vi "ElevatorCtrl_example.vi"() -> ()   [LabVIEW 2019]
uses:
  <vilib>/Rock Robotics/WPI/ThirdParty/JAS_Junk/TrajLib/TypeDef/LINEAR_SYSTEM_LOOP.ctl
  <vilib>/Rock Robotics/WPI/ThirdParty/JAS_Junk/TrajLib/TypeDef/LINEAR_QUADRATIC_REGULATOR.ctl
  <vilib>/Analysis/Matrix/Datatypes/RealMatrix.ctl
  <vilib>/Rock Robotics/WPI/ThirdParty/JAS_Junk/TrajLib/TypeDef/LINEAR_PLANT_INV_FF.ctl
  <vilib>/Rock Robotics/WPI/ThirdParty/JAS_Junk/TrajLib/TypeDef/KALMAN_FILTER.ctl
  <vilib>/Rock Robotics/WPI/ThirdParty/JAS_Junk/TrajLib/TypeDef/LINEAR_SYSTEM.ctl
  <vilib>/Rock Robotics/WPI/ThirdParty/JAS_Junk/TrajLib/Enum/DCMOTOR_TYPES_ENUM.ctl
  <vilib>/Rock Robotics/WPI/ThirdParty/JAS_Junk/TrajLib/BatterySim_CalculateLoadedBatteryVoltage.vi
  <vilib>/Rock Robotics/WPI/ThirdParty/JAS_Junk/TrajLib/Trajectory_Library.lvlib
  <vilib>/Analysis/Matrix/NI_Matrix.lvlib
panel:
  out "out Linear System Loop":T1
  out "Sim Error":bool
  in  "Tab Control":enum32{"Control"}(tab)
  out "Height Dmd \n(SP)":dbl format="%20.3f"
  out "Battery Voltage":dbl format="%20.3f"
  out "CO Chart":cluster{dbl, "Voltage":dbl}(graph)
  in  "GO UP":bool
  out "Elevator\nHeight (PV)":dbl(slide) scale=-1.0..6.0
  out "Height (PV)":dbl format="%20.3f"
  out "Kalman Filtered\nHeight":dbl format="%20.3f"
  out "PV Chart":T7(graph)
  out "Ctrl Error":bool
  out "Motor Dmd (CO)":dbl format="%20.3f"
  out "At Top":bool
  out "At Bottom":bool
  out "Motor Amps":dbl format="%20.3f"
  # "<States,1>"
  # "<FUTURE --- CLAMP TYPE -- For now\nuse Normalize>"
  # "Steady State Gain  \n<States,Outputs>"
  # "State Estimate <Statess,1>"
  # "<States,States>"
  # "<States,Inputs>"
  # "<Outputs,States>"
  # "<Outputs,Inputs>"
  # "<States,1>"
  # "<Inputs,1>"
  # "<States,Inputs>"
  # "<States,States>"
  # "Ref State <States,1>"
  # "Comp and capped \noutput <Inputs,1>"
  # "Controller gain\n<Inputs,States>"
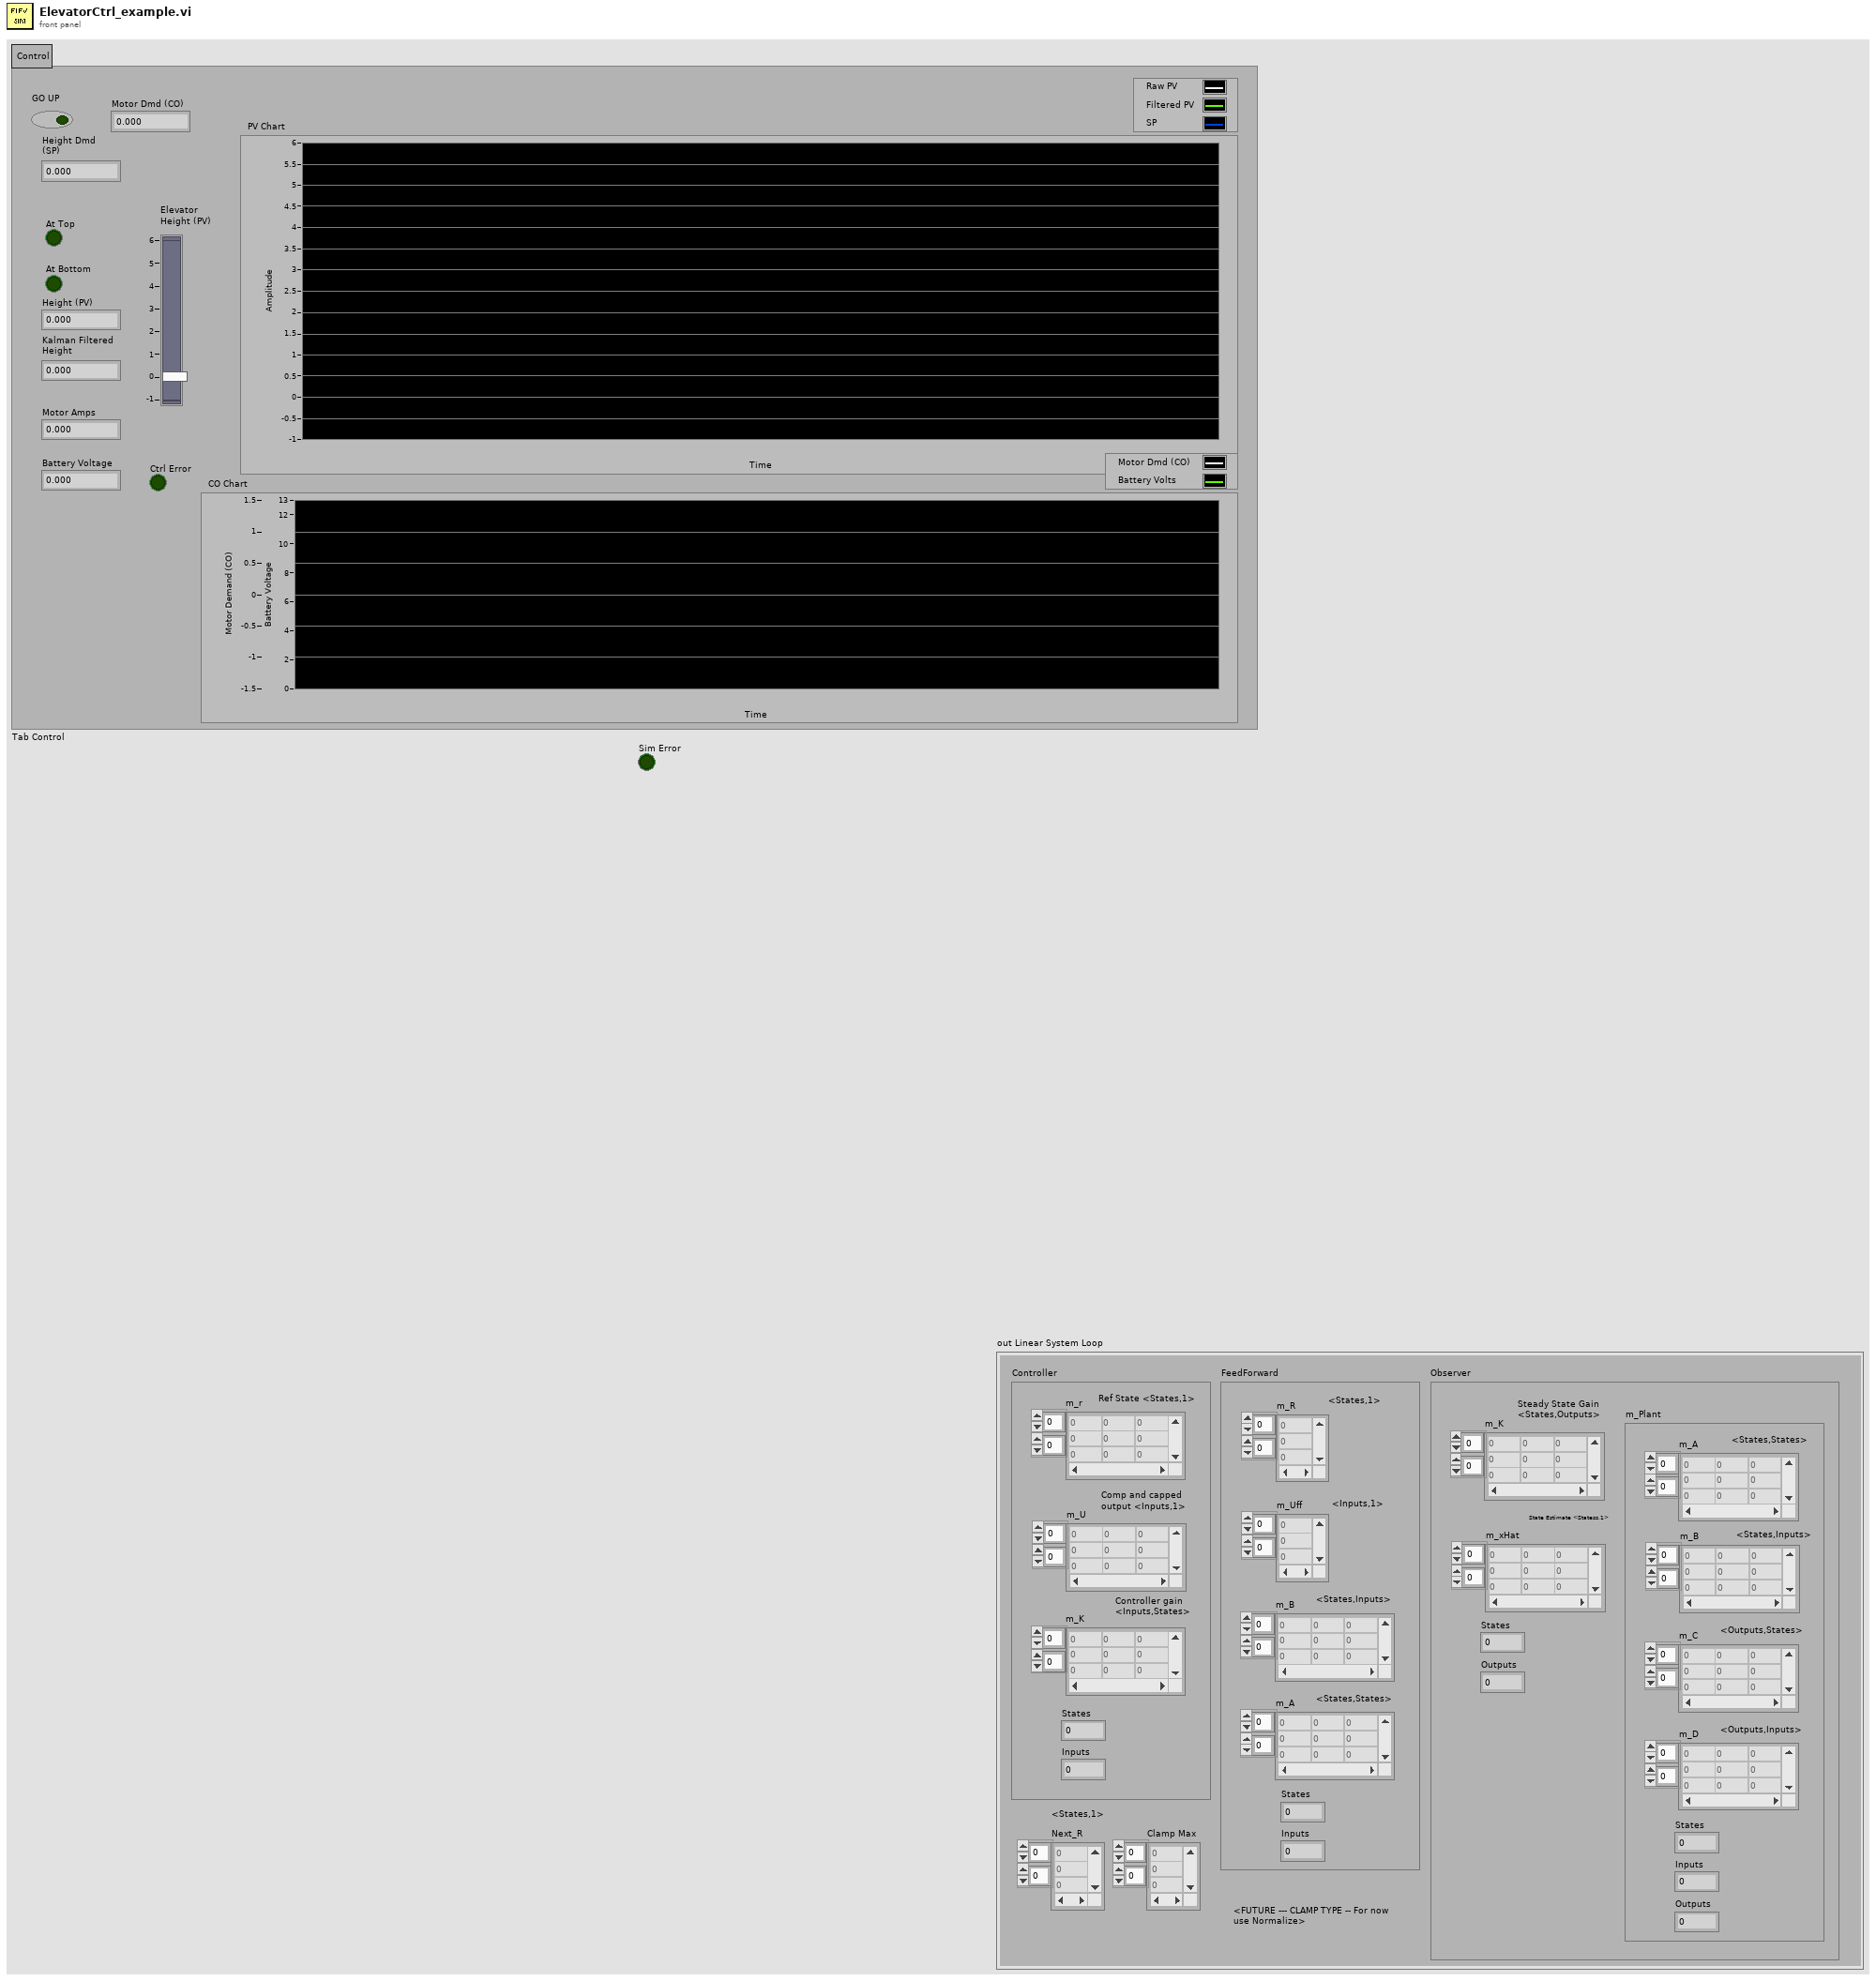
[diagram p1: front panel]
types:
  T1 = typedef "Trajectory_Library.lvlib/LINEAR_SYSTEM_LOOP.ctl" = cluster{"Controller":T2, "FeedForward":T4, "Observer":T5, "Next_R":T3, "Clamp Max":T3}
  T2 = typedef "Trajectory_Library.lvlib/LINEAR_QUADRATIC_REGULATOR.ctl" = cluster{"m_r":T3, "m_U":T3, "m_K":T3, "States":i32, "Inputs":i32}
  T3 = typedef "NI_Matrix.lvlib/RealMatrix.ctl" = dbl[][]
  T4 = typedef "Trajectory_Library.lvlib/LINEAR_PLANT_INV_FF.ctl" = cluster{"m_R":T3, "m_Uff":T3, "m_B":T3, "m_A":T3, "States":i32, "Inputs":i32}
  T5 = typedef "Trajectory_Library.lvlib/KALMAN_FILTER.ctl" = cluster{"m_K":T3, "m_xHat":T3, "States":i32, "Outputs":i32, "m_Plant":T6}
  T6 = typedef "Trajectory_Library.lvlib/LINEAR_SYSTEM.ctl" = cluster{"m_A":T3, "m_B":T3, "m_C":T3, "m_D":T3, "States":i32, "Inputs":i32, "Outputs":i32}
  T7 = cluster{"upper limit":dbl, "Real Matrix Element":dbl, "Real Matrix Element":dbl}
  T8 = typedef "Trajectory_Library.lvlib/DCMOTOR_TYPES_ENUM.ctl" = enum16{"CIM", "AndyMark 9015", "Andy Mark RS 775 125", "Bag", "BaneBots RS 550", "BaneBots RS 775", "Falcon 500", "Mini CIM", "NEO", "NEO 550", "Romi BuiltIn", "Vex 775 Pro", "Snow Blower AM 2235A", "Bosch Seat AM 3493"}
  T9 = typedef "Trajectory_Library.lvlib/LINEAR_SYSTEM_ID_ELEVATOR_MODEL.CTL" = cluster{"DCMOTOR_TYPES":T8, "Num Motors":i32, "WinchRadias_Meters":dbl, "mass_Kg":dbl, "Gearing":dbl}
  T10 = typedef "Trajectory_Library.lvlib/LINEAR_SYSTEM_LOOP_ELEVATOR_CTRL_PARAMS.CTL" = cluster{"Pos Model Std Dev M":dbl, "Vel Model Std Dev M/S":dbl, "Pos Meas Std Dev M":dbl, "Pos Ctrl Tol M":dbl, "Vel Ctrl Tol M/S":dbl, "Max Ctrl Out V":dbl}
  T11 = typedef "Trajectory_Library.lvlib/ELEVATOR_SIM_SIMULATION_PARAMS.ctl" = cluster{"MinHeight_Meters":dbl, "MaxHeight_Meters":dbl, "Measurment StdDev":dbl, "SimulateGravity":bool}
  T12 = cluster{"ElevatorHeight_Meters":dbl, "Kalman Filtered\nHeight":dbl, "f":dbl}
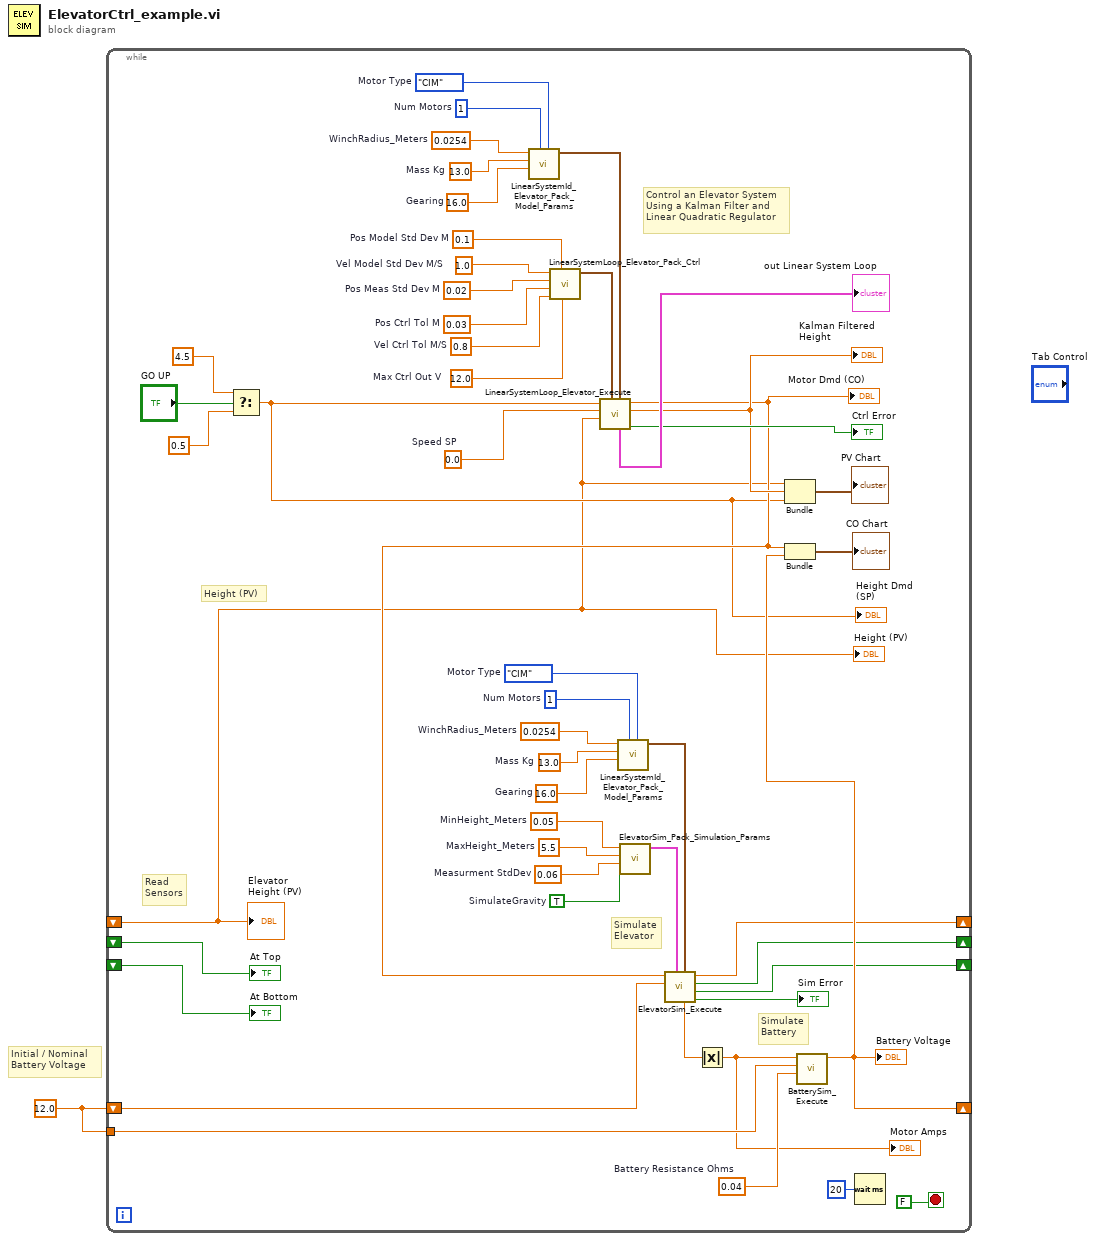
[diagram p0: block diagram]
diagram:
  w1 = 12.0
  # "Initial / Nominal \nBattery Voltage"
  n1 = while {
    shift-right: [w42] -> _
    shift-left: w1 -> [w23]
    tunnel: w1 -> [w43]
    shift-right: [w28] -> _
    shift-left: _ -> [w2]
    shift-right: [w27] -> _
    shift-left: _ -> [w25]
    shift-right: [w26] -> _
    shift-left: _ -> [w24]
    stop <- FALSE stop-if-true
    w8 = 0.0  # Speed SP
    w9 = 1.0  # Vel Model Std Dev M/S
    w10 = 0.02  # Pos Meas Std Dev M
    w11 = 0.03  # Pos Ctrl Tol M
    w12 = 0.8  # Vel Ctrl Tol M/S
    w13 = 0.1  # Pos Model Std Dev M
    w14 = 12.0  # Max Ctrl Out V
    w17 = 0.0254  # WinchRadius_Meters
    w18 = 16.0  # Gearing
    w19 = 13.0  # Mass Kg
    w20 = 1  # Num Motors
    w21 = DCMOTOR_TYPES_ENUM."CIM"  # Motor Type
    w33 = 0.05  # MinHeight_Meters
    w34 = 5.5  # MaxHeight_Meters
    w35 = 0.06  # Measurment StdDev
    w36 = TRUE  # SimulateGravity
    w37 = 0.0254  # WinchRadius_Meters
    w38 = 16.0  # Gearing
    w39 = 13.0  # Mass Kg
    w40 = 1  # Num Motors
    w41 = DCMOTOR_TYPES_ENUM."CIM"  # Motor Type
    w44 = 0.04  # Battery Resistance Ohms
    # "Control an Elevator System\nUsing a Kalman Filter and \nLinear Quadratic Regulator"
    # "Simulate\nBattery"
    # "Simulate\nElevator"
    # "Read\nSensors"
    # "Height (PV)"
    n2 = Select(t=4.5, s="GO UP", f=0.5) -> (s? t:f=w3:dbl)
    "Height Dmd \n(SP)" <- w3
    n3 = call <vilib>:"LinearSystemId_Elevator_Pack_Model_Params.vi"("DCMOTOR_TYPES"=w21, "Num Motors"=w20, "Gearing"=w18, "mass_Kg"=w19, "WinchRadius_Meters"=w17) -> ("Elevator_Model _Params"=w16:T9)  [unwired: 6 in]
    n4 = call <vilib>:"LinearSystemLoop_Elevator_Pack_Ctrl.vi"("Max Ctrl Out V"=w14, "Pos Model Std Dev M"=w13, "Vel Ctrl Tol M/S"=w12, "Pos Ctrl Tol M"=w11, "Pos Meas Std Dev M"=w10, "Vel Model Std Dev M/S"=w9) -> ("LinearSystemLoop_Elevator_Ctrl_Params"=w15:T10)  [unwired: 5 in]
    n5 = call <vilib>:"LinearSystemLoop_Elevator_Execute.vi"("ElevatorSim_Model _Params"=w16, "LinearSystem_Elevator_Ctrl_Params"=w15, "RawHeight PV"=w2, "Speed SP"=w8, "Height SP"=w3) -> ("Error"=→"Ctrl Error":bool, "Kalman Filtered\nHeight"=w5:dbl, "Motor Dmd (CO)"=w4:dbl, "out Linear System Loop"=→"out Linear System Loop":T1)  [unwired: 3 in]
    "Kalman Filtered\nHeight" <- w5
    "Motor Dmd (CO)" <- w4
    n6 = call <vilib>:"LinearSystemId_Elevator_Pack_Model_Params.vi"("DCMOTOR_TYPES"=w41, "Num Motors"=w40, "Gearing"=w38, "mass_Kg"=w39, "WinchRadius_Meters"=w37) -> ("Elevator_Model _Params"=w32:T9)  [unwired: 6 in]
    n7 = call <vilib>:"ElevatorSim_Pack_Simulation_Params.vi"("SimulateGravity"=w36, "Measurment StdDev"=w35, "MaxHeight_Meters"=w34, "MinHeight_Meters"=w33) -> ("ElevatorSim_Simulation _Params"=w31:T11)  [unwired: 7 in]
    n8 = call <vilib>:"ElevatorSim_Execute.vi"("LinearSystemID_Elevator_Model _Params"=w32, "ElevatorSim_Simulation _Params"=w31, "Battery Volts"=w23, "Motor Dmd"=w4) -> ("Error"=→"Sim Error":bool, "AtLowLimit"=w26:bool, "At HIgh LImit"=w27:bool, "ElevatorHeight_Meters"=w28:dbl, "Motor Current"=w30:dbl)  [unwired: 2 in, 1 out]
    n9 = Absolute Value(x=w30) -> (abs(x)=w29:dbl)
    "Motor Amps" <- w29
    n10 = Bundle("ElevatorHeight_Meters"=w2, "Kalman Filtered\nHeight"=w5, "f"=w3) -> (→"PV Chart":T12)  [unwired: 1 in]
    n11 = call <vilib>:"BatterySim_Execute.vi"("Battery Resistance Ohms"=w44, "Nominal Battery Voltage"=w43, "Current"=w29) -> ("Voltage"=w42:dbl)  [unwired: 8 in]
    "Battery Voltage" <- w42
    n12 = Bundle("Motor Dmd (CO)"=w4, "Voltage"=w42) -> (→"CO Chart":cluster{"Motor Dmd (CO)":dbl, "Voltage":dbl})  [unwired: 1 in]
    n13 = Wait (ms)(milliseconds to wait=u32 20) -> ()  [unwired: 1 out]
    "Elevator\nHeight (PV)" <- w2
    "Height (PV)" <- w2
    "At Top" <- w25
    "At Bottom" <- w24
  }
